vi "Main.vi"() -> ()   [LabVIEW 2015]
uses:
  <vilib>/Instr/_visa.llb/Select Event Type.ctl
  <vilib>/Instr/_visa.llb/VISA Configure Serial Port (Instr).vi
panel:
  out "Input Waveform":T1(graph)
  out "Loop period (ms)":u32
  out "Bytes Remaining":u32
  out "Arduino Sample Rate (S/s)":dbl format="%.2f"
  out "Loop Iterations":i32
  out "Error Out":errorcluster
  out "Serial Monitor":string
  in  "Stop":bool
  out "New Serial Data":string
  in  "COM Port":refnum<visa-resource-name>="COM71"
  # "Arduino Labview Voltage Display"
  # "Created by zxlee (iamzxlee.wordpress.com)"
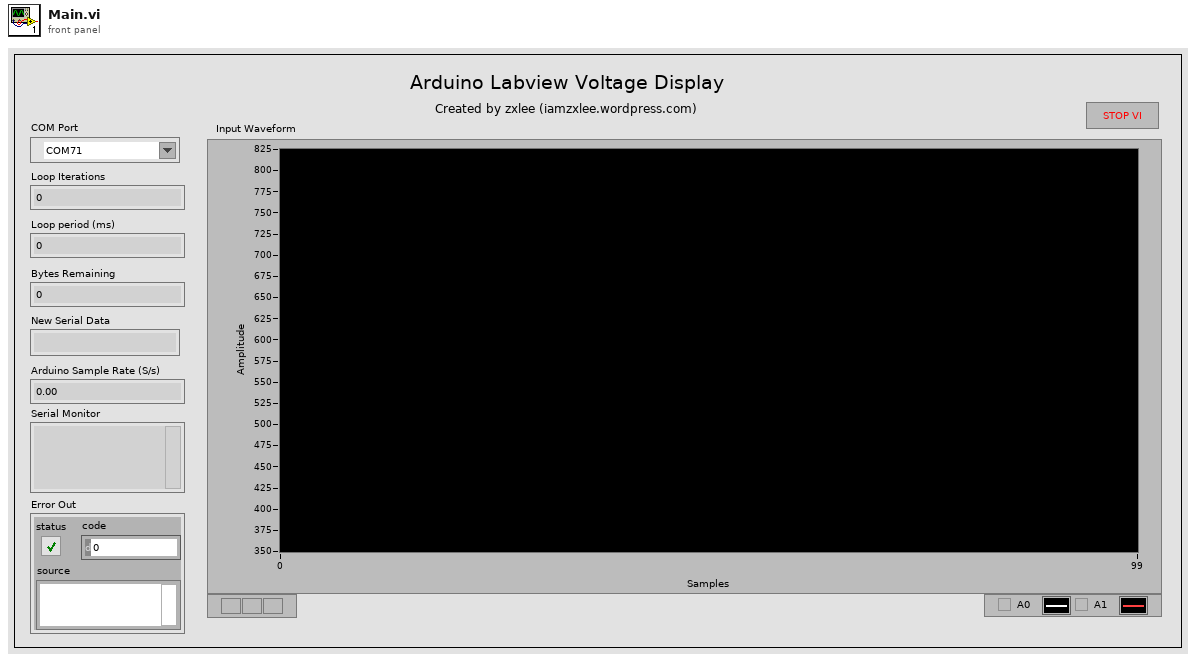
[diagram p1: front panel]
types:
  T1 = cluster{"default value 1":i16, "default value 1":i16}
  T2 = cluster{"default value 1":i16, "default value 1":i16}[]
  T3 = typedef "Select Event Type.ctl" = u32
  T4 = cluster{"baud rate (9600)":u32, "data bits (8)":u16, "parity (0:none)":enum16{"None", "Odd", "Even", "Mark", "Space"}, "stop bits (10: 1 bit)":u16, "flow control (0:none)":u16}
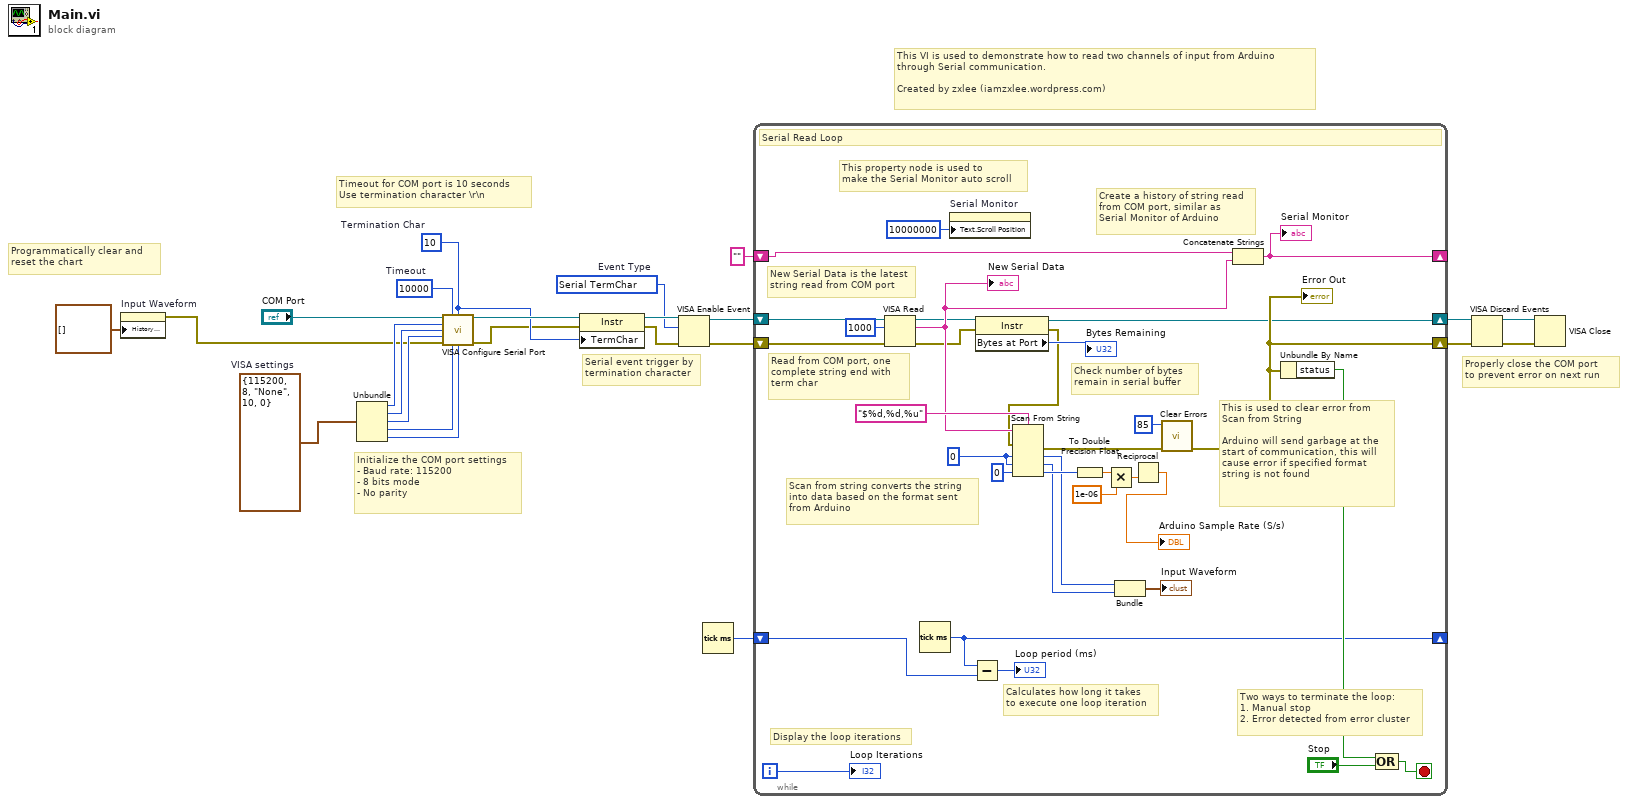
[diagram p0: block diagram]
diagram:
  w5 = T3 1073684516 items=["Service Request"=1073684491, "Trigger"=3221168138, "Clear"=1073684493, "VXI Signal"=1073684512, "VXI/VME Interrupt"=3221168161, "VXI/VME Sysfail"=1073684509, "VXI/VME Sysreset"=1073684510, "GPIB CIC"=1073684498, "GPIB Talk"=1073684499, "GPIB Listen"=1073684500, "PXI Interrupt"=1073684514, "Serial Break"=1073684515, "Serial TermChar"=1073684516, "Serial CTS"=1073684521, "Serial DSR"=1073684522, "Serial DCD"=1073684524, "Serial RI"=1073684526, "Serial Character"=1073684533, "USB Interrupt"=1073684535, "All Enabled"=1073709055]  # Event Type
  w15 = u8 10  # Termination Char
  w17 = u32 10000  # Timeout
  w23 = T4 {"baud rate (9600)"=115200, "data bits (8)"=8, "parity (0:none)"=enum."None", "stop bits (10: 1 bit)"=10, "flow control (0:none)"=0}  # VISA settings
  # "Programmatically clear and \nreset the chart"
  # "This VI is used to demonstrate how to read two channels of input from Arduino\nthrough Serial communication.\n\nCreated by zxlee (iamzxlee.wordpress.com)"
  # "Properly close the COM port \nto prevent error on next run"
  # "Serial event trigger by\ntermination character"
  # "Timeout for COM port is 10 seconds\nUse termination character \\r\\n"
  # "Initialize the COM port settings\n- Baud rate: 115200\n- 8 bits mode\n- No parity"
  n1 = property on="Input Waveform" class="WFChart (strict)"("History Data"=T2 []) -> (error out=w1:errorcluster)  [unwired: 2 in, 1 out]
  n2 = Unbundle(w23) -> ("baud rate (9600)"=w22:u32, "data bits (8)"=w21:u16, "parity (0:none)"=w20:enum16{"None", "Odd", "Even", "Mark", "Space"}, "stop bits (10: 1 bit)"=w19:u16, "flow control (0:none)"=w18:u16)
  n3 = call-poly "VISA Configure Serial Port"("VISA resource name"="COM Port", "timeout (10sec)"=w17, "termination char\n(0xA = '\\n' = LF)"=w15, "baud rate (9600)"=w22, "data bits (8)"=w21, "parity (0:none)"=w20, "error in (no error)"=w1, "stop bits (10: 1 bit)"=w19, "flow control (0:none)"=w18) -> ("VISA resource name out"=w16:refnum<visa-resource-name>, "error out"=w14:errorcluster)  [unwired: 5 in]
  n4 = property class="Instr"(reference=w16, error in=w14, "TermChar"=w15) -> (reference out=w13:refnum<visa-resource-name>, error out=w12:errorcluster)
  n5 = VISA Enable Event(8:w12, 10:w5, 11:w13) -> (0:w10:errorcluster, 3:w11:refnum<visa-resource-name>)  [unwired: 1 in]
  n6 = Tick Count (ms)() -> (millisecond timer value=w3:u32)
  n7 = while {
    shift-right: [w49] -> w6
    shift-left: w10 -> [w56]
    shift-right: [w25] -> w7
    shift-left: w11 -> [w57]
    shift-right: [w54] -> _
    shift-left: "" -> [w53]
    shift-right: [w42] -> _
    shift-left: w3 -> [w41]
    i -> [w51]
    stop <- w47 stop-if-true
    w39 = i16 0 ("default value 1")
    # "Calculates how long it takes\nto execute one loop iteration"
    # "Check number of bytes\nremain in serial buffer"
    # "This property node is used to \nmake the Serial Monitor auto scroll"
    # "Two ways to terminate the loop:\n1. Manual stop\n2. Error detected from error cluster"
    # "Display the loop iterations"
    # "This is used to clear error from \nScan from String\n\nArduino will send garbage at the\nstart of communication, this will\ncause error if specified format \nstring is not found"
    # "Scan from string converts the string\ninto data based on the format sent\nfrom Arduino"
    # "Create a history of string read\nfrom COM port, similar as\nSerial Monitor of Arduino"
    # "New Serial Data is the latest\nstring read from COM port"
    # "Read from COM port, one\ncomplete string end with\nterm char"
    # "Serial Read Loop"
    n8 = VISA Read(VISA resource name=w57, byte count=u32 1000, error in (no error)=w56) -> (VISA resource name out=w28:refnum<visa-resource-name>, read buffer=w48:string, error out=w27:errorcluster)  [unwired: 1 out]
    "New Serial Data" <- w48
    n9 = Tick Count (ms)() -> (millisecond timer value=w42:u32)
    n10 = property on="Serial Monitor" class="Str"("Text.Scroll Position"=u32 10000000) -> ()  [unwired: 2 in, 2 out]
    n11 = Subtract(x=w42, y=w41) -> (x-y=→"Loop period (ms)":u32)
    n12 = property class="Instr"(reference=w28, error in=w27) -> (reference out=w25:refnum<visa-resource-name>, error out=w26:errorcluster, "Bytes at Port"=→"Bytes Remaining":u32)
    n13 = Scan From String(format string="$%d,%d,%u", input string=w48, error in=w26, default 1=w39, default 2=w39, default 3=u32 0 ("default value 3")) -> (error out=w37:errorcluster, output 1=w31:i16, output 2=w30:i16, output 3=w35:u32)  [unwired: 1 in, 2 out]
    n14 = To Double Precision Float(number=w35) -> (double precision float=w33:dbl)
    n15 = Multiply(x=w33, y=1e-06) -> (x*y=w34:dbl)
    n16 = Bundle("default value 1"=w31, "default value 1"=w30) -> (→"Input Waveform":T1)  [unwired: 1 in]
    n17 = Reciprocal(x=w34) -> (1/x=→"Arduino Sample Rate (S/s)":dbl)
    n18 = call <vilib>:"Clear Errors.vi"("error in (no error)"=w37, "specific error code to clear (0: all)"=85) -> ("error out"=w49:errorcluster)  [unwired: 4 in, 1 out]
    "Error Out" <- w49
    n19 = Concatenate Strings(w53, w48) -> (w54:string)
    "Serial Monitor" <- w54
    n20 = Unbundle By Name(w49) -> ("status"=w45:bool)
    n21 = Compound Arithmetic op=OR(w45, "Stop") -> (w47:bool)
    "Loop Iterations" <- w51
  }
  n22 = VISA Discard Events(8:w6, 11:w7) -> (0:w8:errorcluster, 3:w9:refnum<visa-resource-name>)  [unwired: 2 in]
  n23 = VISA Close(VISA resource name=w9, error in (no error)=w8) -> ()  [unwired: 1 out]
